vi "Split Nested Members.vi"(5 "Root TypeID":string, 10 "Item Graph":T1[](array[typedef]), 11 "Member Index":i32) -> (2 "TypeIDs":string[](array[string]), 3 "Names":string[](array[string]))   [LabVIEW 2020, in "Better Search.lvlib"]
uses:
  Better Search.lvlib
  Data Types/Type Reflection Item.ctl
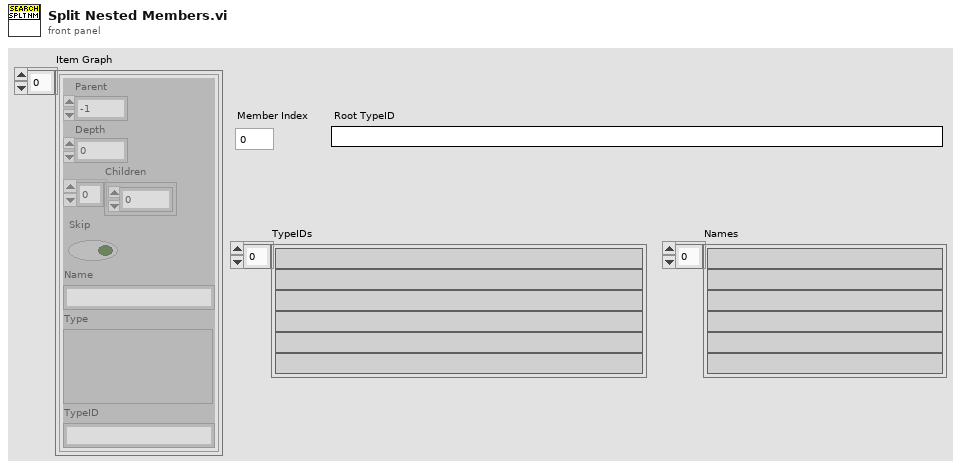
[diagram p1: front panel]
types:
  T1 = typedef "Better Search.lvlib/Type Reflection Item.ctl" = cluster{"Parent":i32, "Depth":i32, "Children":i32[], "Skip":bool, "Name":string, "Type":variant, "TypeID":string}
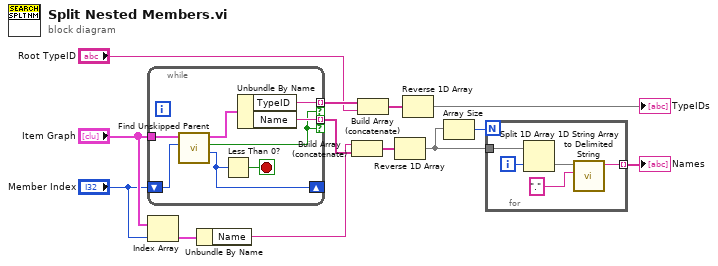
[diagram p0: block diagram]
diagram:
  n1 = while {
    shift-right: [w15] -> _
    shift-left: "Member Index" -> [w20]
    tunnel: "Item Graph" -> [w21]
    tunnel: [w18] -> w11 mode=indexing if=w16
    tunnel: [w17] -> w13 mode=indexing if=w16
    stop <- w14 stop-if-true
    n2 = call "Find Unskipped Parent.vi"("Start Index"=w20, "Graph In"=w21) -> ("Index"=w15:i32, "Found?"=w16:bool, "Unskipped Parent"=w19:T1)  [unwired: 7 in]
    n3 = Less Than 0?(x=w15) -> (x < 0?=w14:bool)
    n4 = Unbundle By Name(w19) -> ("TypeID"=w17:string, "Name"=w18:string)
  }
  n5 = Index Array(array="Item Graph", index="Member Index") -> (element=w8:T1)
  n6 = Unbundle By Name(w8) -> ("Name"=w7:string)
  n7 = Build Array (concatenate)(w7, w11) -> (w6:string[])
  n8 = Build Array (concatenate)(w13, "Root TypeID") -> (w2:string[])
  n9 = Reverse 1D Array(array=w6) -> (reversed array=w4:string[])
  n10 = Reverse 1D Array(array=w2) -> (reversed array=→"TypeIDs":string[])
  n11 = Array Size(array=w4) -> (size(s)=w3:i32)
  n12 = for {
    N: w3 -> [_]
    tunnel: w4 -> [w26]
    tunnel: [w22] -> w5 mode=indexing
    i -> [w25]
    n13 = Split 1D Array(array=w26, index=w25) -> (second subarray=w24:string[])  [unwired: 1 out]
    n14 = call <vilib>:"1D String Array to Delimited String.vi"("delimiter"=".", "string array"=w24) -> ("delimited string"=w22:string)  [unwired: 9 in]
  }
  "Names" <- w5
